vi "Check Action.vi"(6 "HRS Time":dbl, 7 "Values In":dbl[](array[numeric]), 8 "error in (no error)":errorcluster, 11 "Valve in":refnum<class "HitAndHoldControl.lvclass">) -> (0 "error out":errorcluster, 2 "Actions":T1[](array[typedef]), 3 "Valve out":refnum<class "HitAndHoldControl.lvclass">, 5 "Values":dbl[](array[numeric]))   [LabVIEW 2023, in "VolatusControl.lvlib" / "HitAndHoldControl.lvclass"]
uses:
  HitAndHoldControl.lvclass
  Control Action.ctl
  Volatus/MessageQ/MessageQ.lvclass
  HitAndHoldControl.lvclass/HitAndHoldControl.ctl
  HitAndHold State.ctl
  messages/CmdAnalog/Data.ctl
  Volatus/MessageQ/MessageQ.lvclass/MessageQ.ctl
  messages/CmdAnalog/CmdAnalog.lvlib
  messages/CmdAnalogMultiple/CmdAnalogMultiple.lvlib
  VolatusControl.lvlib
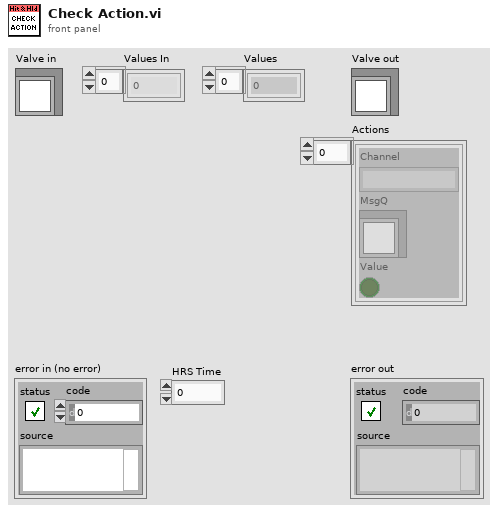
[diagram p1: front panel]
types:
  T1 = typedef "VolatusControl.lvlib/Control Action.ctl" = cluster{"Channel":string, "MsgQ":refnum<class "MessageQ.lvclass">, "Value":bool}
  T2 = typedef "VolatusControl.lvlib/HitAndHoldControl.lvclass/HitAndHold State.ctl" = enum16{"Idle", "Hit", "Dwell", "Hold", "Off"}
  T3 = typedef "CmdAnalog.lvlib/Data.ctl" = cluster{"channel":string, "value":dbl}
  T4 = typedef "CmdAnalogMultiple.lvlib/Data.ctl" = cluster{"values":T3[]}
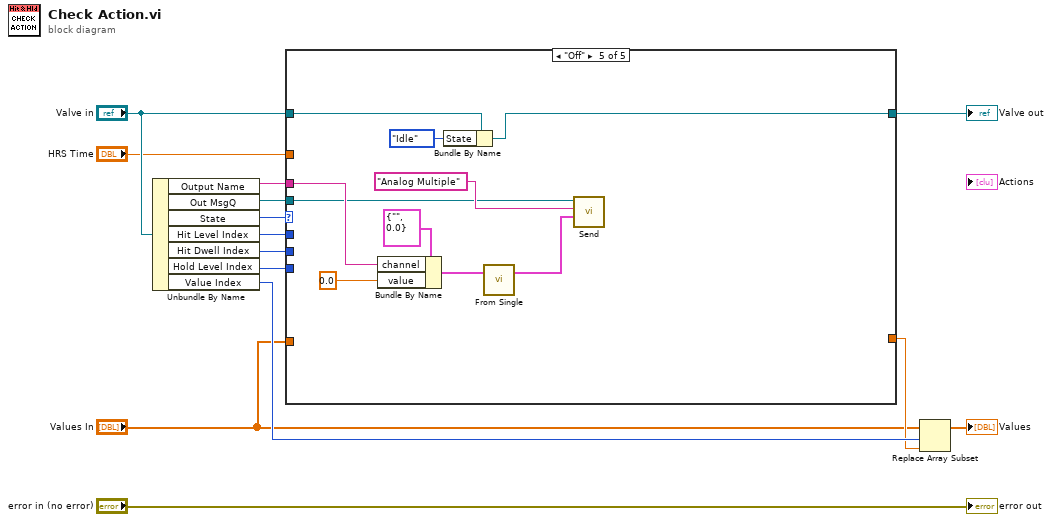
[diagram p0: block diagram]
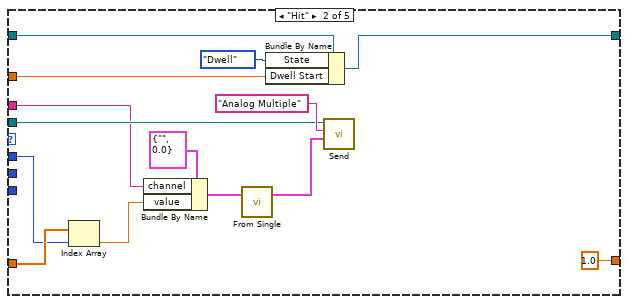
[diagram p3: hidden frame]
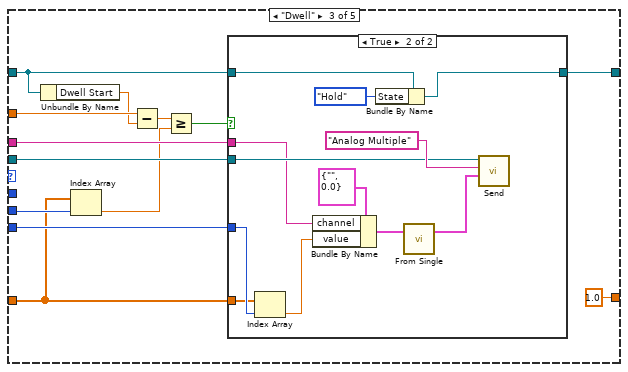
[diagram p4: hidden frame]
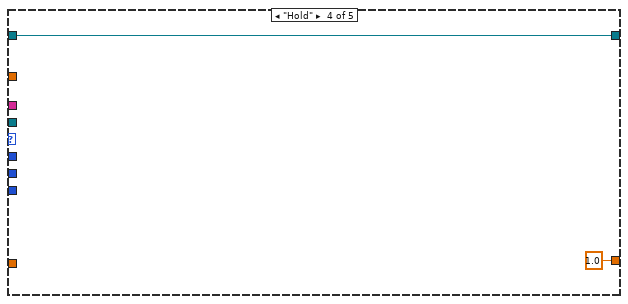
[diagram p6: hidden frame]
diagram:
  n1 = Unbundle By Name("Valve in") -> ("Output Name"=w4:string, "Out MsgQ"=w11:refnum<class "MessageQ.lvclass">, "State"=w12:T2, "Hit Level Index"=w10:i32, "Hit Dwell Index"=w9:i32, "Hold Level Index"=w8:i32, "Value Index"=w6:i32)
  n2 = case shown="\"Off\"" w12 {
    tunnel: "Valve in" -> [w15 w28 w40 w56 w61]
    tunnel: w11 -> [_ w21 w38 _ w63]
    tunnel: w10 -> [_ w18 _ _ _]
    tunnel: w9 -> [_ _ w41 _ _]
    tunnel: w8 -> [_ _ w36 _ _]
    tunnel: [_ 1.0 1.0 1.0 _] -> w5
    tunnel: w4 -> [_ w20 w37 _ w64]
    tunnel: "Values In" -> [_ w19 w35 _ _]
    tunnel: "HRS Time" -> [_ w25 w34 _ _]
    tunnel: [w15 w27 w39 w56 w60] -> w1
    frame "Idle" {
    }
    frame "Hit" {
      n3 = Index Array(array=w19, index=w18) -> (element=w17:dbl)
      n4 = Bundle By Name(cluster=T3 {"channel"="", "value"=0.0} ("CmdAnalog"), "channel"=w20, "value"=w17) -> (w23:T3)
      n5 = call "From Single.vi"("CmdAnalog"=w23) -> ("CmdAnalogMultiple"=w16:T4)  [unwired: 6 in]
      n6 = Bundle By Name(cluster=w28, "State"=HitAndHold_State."Dwell", "Dwell Start"=w25) -> (w27:refnum<class "HitAndHoldControl.lvclass">)
      n7 = call "Send.vi"("Data"=w16, "ID"="Analog Multiple", "MessageQ in"=w21) -> ()  [unwired: 7 in, 2 out]
    }
    frame "Dwell" {
      n8 = Unbundle By Name(w40) -> ("Dwell Start"=w33:dbl)
      n9 = Index Array(array=w35, index=w41) -> (element=w31:dbl)
      n10 = Subtract(x=w34, y=w33) -> (x-y=w32:dbl)
      n11 = Greater Or Equal?(x=w32, y=w31) -> (x >= y?=w30:bool)
      n12 = case shown="True" w30 {
        tunnel: w40 -> [w43 w55]
        tunnel: [w43 w54] -> w39
        tunnel: w38 -> [_ w47]
        tunnel: w37 -> [_ w46]
        tunnel: w36 -> [_ w52]
        tunnel: w35 -> [_ w51]
        frame False {
        }
        frame True {
          n13 = Index Array(array=w51, index=w52) -> (element=w45:dbl)
          n14 = Bundle By Name(cluster=T3 {"channel"="", "value"=0.0} ("CmdAnalog"), "channel"=w46, "value"=w45) -> (w49:T3)
          n15 = Bundle By Name(cluster=w55, "State"=HitAndHold_State."Hold") -> (w54:refnum<class "HitAndHoldControl.lvclass">)
          n16 = call "From Single.vi"("CmdAnalog"=w49) -> ("CmdAnalogMultiple"=w44:T4)  [unwired: 6 in]
          n17 = call "Send.vi"("Data"=w44, "ID"="Analog Multiple", "MessageQ in"=w47) -> ()  [unwired: 7 in, 2 out]
        }
      }
    }
    frame "Hold" {
    }
    frame "Off" {
      n18 = Bundle By Name(cluster=T3 {"channel"="", "value"=0.0} ("CmdAnalog"), "channel"=w64, "value"=0.0) -> (w66:T3)
      n19 = Bundle By Name(cluster=w61, "State"=HitAndHold_State."Idle") -> (w60:refnum<class "HitAndHoldControl.lvclass">)
      n20 = call "From Single.vi"("CmdAnalog"=w66) -> ("CmdAnalogMultiple"=w58:T4)  [unwired: 6 in]
      n21 = call "Send.vi"("Data"=w58, "ID"="Analog Multiple", "MessageQ in"=w63) -> ()  [unwired: 7 in, 2 out]
    }
  }
  "Valve out" <- w1
  n22 = Replace Array Subset(array="Values In", new element=w5, index=w6) -> (→"Values":dbl[])
  "error out" <- "error in (no error)"
